vi "HTML Report.vi"() -> ()   [LabVIEW 2023]
doc: "This is an example of some of the things that you can do with HTML reports."
uses:
  <vilib>/Utility/NIReport.llb/image depth.ctl
  <vilib>/Utility/NIReport.llb/Report Type.ctl
  <vilib>/Utility/NIReport.llb/Append Report Text (str wrap).vi
  <vilib>/printing/OpenHTMLReport.llb/Open HTML Report in Browser (Refnum).vi
  <vilib>/Utility/NIReport.llb/NI_report.lvclass
  <vilib>/Utility/NIReport.llb/NI_ReportGenerationCore.lvlib
panel:
  out "Temporary HTML file created":path
  out "Waveform Graph":dbl[](graph)=[0.5636359789434375, 0.46587763826260464, 0.8325692892892249, 0.8300180783614736, 0.9824977234810706, 0.9246798162864311, 0.28797705040319066, 0.8866968704790259, 0.02130389365515839, 0.877123252962531, 0.9643395004283489, 0.02059887842576158, 0.1273108305149826, 0.41136455122560744, 0.2854242872286874, 0.9465048697296147, 0.7783839826944587, 0.8639156271001904, 0.9978296411706133, 0.5287970384773009, 0.35322400657448116, 0.18914478038148386, 0.8592356514211328, 0.7912972224138053, 0.5333597681988271, 0.06514822279027666, 0.7994102766311608, 0.340457166877981, 0.506120264737175, 0.4156698088803017, 0.8094252612693209, 0.4166808970347642, 0.02572497487244574, 0.7986194804518524, 0.19795741292293068, 0.9574498541610317, 0.29863723910280027, 0.7677081160903261, 0.347174302983873, 0.35006132052667427, 0.04602735268300018, 0.9347641692596718, 0.5276729641187805, 0.9182839031881829, 0.788749036568972, 0.8552127532811189, 0.3284535717394679, 0.25634529864403, 0.8758337995990879, 0.177291751844876, 0.8051323605071565, 0.6771930271702604, 0.4299889818646203, 0.8654484701471663, 0.7051704458851662, 0.9906228655515175, 0.19635072646547425, 0.7451544322796311, 0.938468964228471, 0.48382664446866963, 0.796164009209664, 0.5511315678287445, 0.2066875319208923, 0.5599194900492128, 0.07942966626324477, 0.417018433935066, 0.048298330540019974, 0.5944847894375902, 0.9949580369525495, 0.6034072336020191, 0.565572814588545, 0.03259207285515475, 0.8455914772729686, 0.4424681502033191, 0.6785504027661995, 0.11530841686781357, 0.8045290001921432, 0.7942797286449228, 0.2692216813705599, 0.48648707714837003, 0.31795114769939015, 0.6652772141956849, 0.8218573324475937, 0.6215707304190634, 0.5789347292932601, 0.10243357286355437, 0.7510243492947337, 0.4014679232179792, 0.5567364642901194, 0.824093293491236, 0.3985459275229004, 0.9330783494704211, 0.8545270337950668, 0.4528476949522773, 0.5608950239830195, 0.38370738497260515, 0.597263836832918, 0.3728397850091074, 0.36167347648435544, 0.3615909297962516]
  in  "Header":string="Example Report with Images"
  in  "Body":string="<tab>This is an example of some of the things that you can do with HTML reports. <newline> <tab>Above is an image of a Waveform Chart Control.  Below is a horizontal line.  Below that is a link to NI's homepage.<newline>"
  # "Overview: Demonstrates generating and displaying an HTML report.\nInstructions:\n1. Run the VI.\n2. The generated report will be displayed in your default web browser.\n3. Delete the temporary HTML file (located at the path indicated by Temporary HTML file created) when you are done."
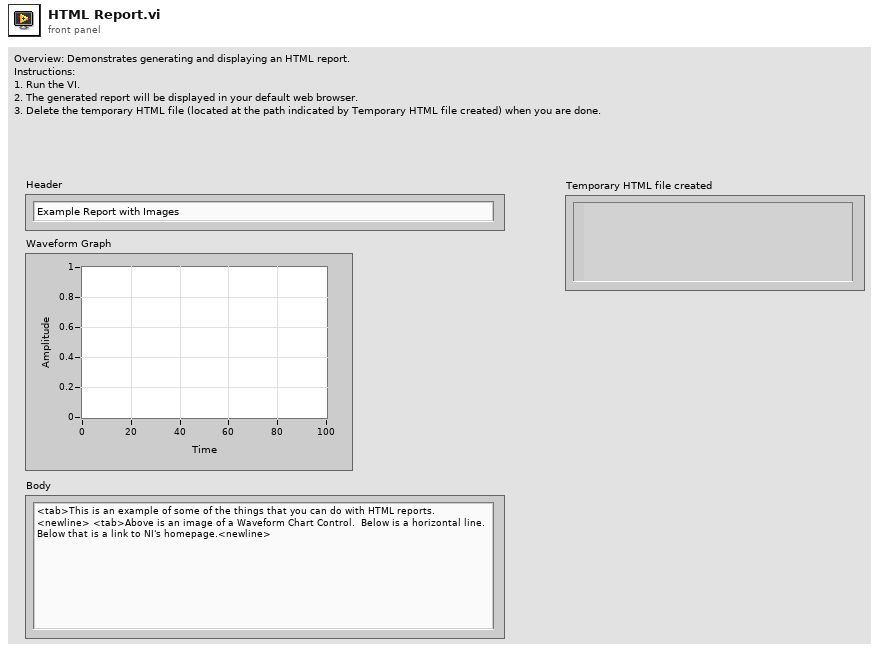
[diagram p1: front panel]
types:
  T1 = typedef "NI_ReportGenerationCore.lvlib/Report Type.ctl" = enum16{"HTML", "Word", "Excel"}
  T2 = typedef "NI_ReportGenerationCore.lvlib/image depth.ctl" = u16
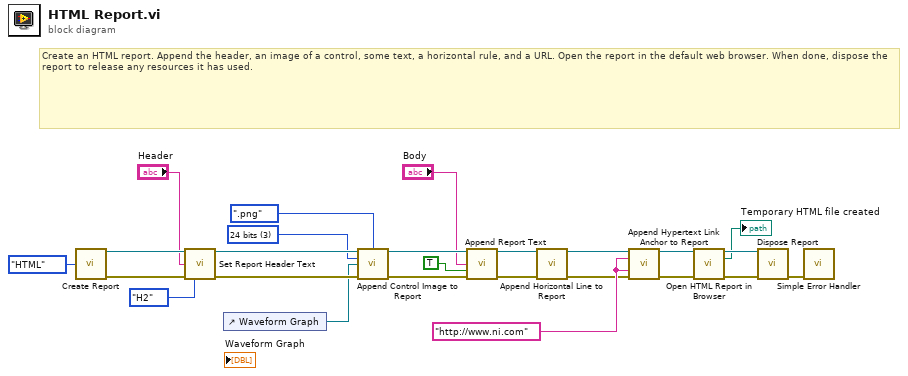
[diagram p0: block diagram]
diagram:
  w5 = T2 3 items=["B&W", "4 bits", "8 bits", "24 bits"] ("image depth")
  w24 = "http://www.ni.com" ("URL of link - href")
  # "Create an HTML report. Append the header, an image of a control, some text, a horizontal rule, and a URL. Open the report in the default web browser. When done, dispose the report to release any resources it has used."
  n1 = call <vilib>:"Create Report.vi"("report type"=Report_Type."HTML" ("Report Type")) -> ("report out"=w22:refnum<class "NI_report.lvclass">, "error out"=w23:errorcluster)  [unwired: 13 in]
  n2 = call-dynamic "Set Report Header Text.vi"("report in"=w22, "center header text"="Header", "error in (no error)"=w23, "HTML header size"=enum16{"H1", "H2", "H3", "H4", "H5", "H6", "H7"}."H2") -> ("report out"=w13:refnum<class "NI_report.lvclass">, "error out"=w10:errorcluster)  [unwired: 10 in]
  n3 = control-ref of="Waveform Graph"() -> (w9:refnum<vi>)
  n4 = call-dynamic "Append Control Image to Report.vi"("report in"=w13, "image file type (.jpg)"=enum16{".jpg", ".png"}.".png" ("image file type"), "image depth"=w5, "ctrl reference"=w9, "error in (no error)"=w10) -> ("report out"=w16:refnum<class "NI_report.lvclass">, "error out"=w17:errorcluster)  [unwired: 7 in, 2 out]
  n5 = call-poly <vilib>:"Append Report Text.vi"("report in"=w16, "text"="Body", "append on new line? (F)"=TRUE, "error in (no error)"=w17) -> ("report out"=w15:refnum<class "NI_report.lvclass">, "error out"=w14:errorcluster)  [unwired: 8 in, 2 out]
  n6 = call-dynamic "Append Horizontal Line to Report.vi"("report in"=w15, "error in (no error)"=w14) -> ("report out"=w8:refnum<class "NI_report.lvclass">, "error out"=w7:errorcluster)  [unwired: 12 in]
  n7 = call-dynamic "Append Hypertext Link Anchor to Report.vi"("report in"=w8, "URL of link - href"=w24, "link text"=w24, "error in (no error)"=w7) -> ("report out"=w2:refnum<class "NI_report.lvclass">, "error out"=w3:errorcluster)  [unwired: 8 in, 2 out]
  n8 = call-poly <vilib>:"Open HTML Report in Browser.vi"("report in"=w2, "error in (no error)"=w3) -> ("report out"=w6:refnum<class "NI_report.lvclass">, "temporary HTML file created"=→"Temporary HTML file created":path, "error out"=w25:errorcluster)  [unwired: 11 in]
  n9 = call-dynamic "Dispose Report.vi"("report in"=w6, "error in (no error)"=w25) -> ("error out"=w12:errorcluster)  [unwired: 13 in]
  n10 = call <vilib>:"Simple Error Handler.vi"("error in (no error)"=w12) -> ()  [unwired: 4 in, 5 out]
